vi "UnitConv(Time).vi"(5 "Unit IN":string, 6 "precision (0)":i16, 7 "Num IN":dbl format="%.1e", 8 "St IN":string) -> (1 "St OUT":string, 2 "NumOUT":dbl format="%.1e", 4 "Unit OUT":string)   [LabVIEW 2017]
panel:
  in  "Mult 2":dbl[](array[numeric])=[1e-09, 1e-06, 0.001, 1.0, 60.0, 3600.0, 86400.0] format="%.1e"
  in  "Unit 2":string[](array[string])=["ns", "us", "ms", "s", "min", "h", "day"]
  in  "Mult":dbl[](array[numeric])=[1.0, 1e-09, 1e-06, 0.001, 1.0, 60.0, 3600.0, 86400.0] format="%.1e"
  in  "Unit":string[](array[string])=["ns", "us", "ms", "s", "min", "h", "day"]
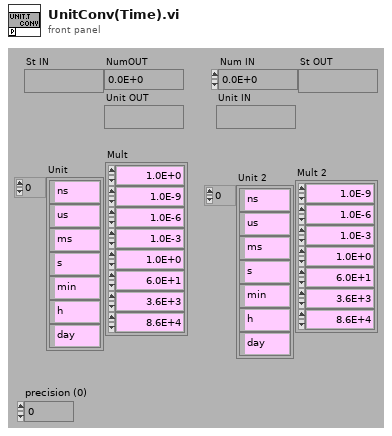
[diagram p1: front panel]
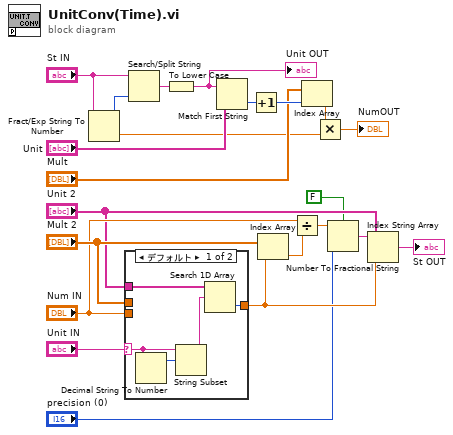
[diagram p0: block diagram]
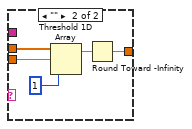
[diagram p2: hidden frame]
diagram:
  n1 = Fract/Exp String To Number(string="St IN") -> (offset past number=w22:i32, number=w15:dbl)  [unwired: 3 out]
  n2 = case shown="デフォルト" "Unit IN" {
    selector: "Unit IN" -> [w24 _]
    tunnel: "Mult 2" -> [_ w32]
    tunnel: "Num IN" -> [_ w28]
    tunnel: [w27 w31] -> w7
    tunnel: "Unit 2" -> [w26 _]
    frame Default {
      n3 = Decimal String To Number(string=w24) -> (offset past number=w25:i32)  [unwired: 3 out]
      n4 = String Subset(string=w24, offset (0)=w25) -> (substring=w23:string)  [unwired: 1 out]
      n5 = Search 1D Array(1D array=w26, element=w23) -> (index of element=w27:i32)  [unwired: 1 out]
    }
    frame "" {
      n6 = Threshold 1D Array(1:1 ("start index (0)"), 2:w28, 3:w32) -> (0:w30:dbl)
      n7 = Round Toward -Infinity(1:w30) -> (0:w31:dbl)
    }
  }
  n8 = Search/Split String(string="St IN", offset (0)=w22) -> (match + rest of string=w4:string)  [unwired: 3 out]
  n9 = To Lower Case(string=w4) -> (all lower case string=w3:string)
  "Unit OUT" <- w3
  n10 = Match First String(2:"Unit", 3:w3) -> (0:w19:i32)  [unwired: 1 out]
  n11 = Increment(x=w19) -> (x+1=w18:i32)
  n12 = Index Array(array="Mult 2", index=w7) -> (element=w12:dbl)
  n13 = Divide(x="Num IN", y=w12) -> (x/y=w10:dbl)
  n14 = Index Array(array="Mult", index=w18) -> (element=w16:dbl)
  n15 = Multiply(x=w16, y=w15) -> (x*y=→"NumOUT":dbl)
  n16 = Number To Fractional String(use system decimal point (T)=FALSE, number=w10, precision (6)="precision (0)") -> (F-format string=w9:string)  [unwired: 1 out]
  n17 = Index String Array(1:w7, 2:"Unit 2", 3:w9) -> (0:→"St OUT":string)
